vi "CD Init_Prepare Inline Data_Compute Index from CWD1 FOR Broadcast.vi"(11 "message":T1 {"Timestamp Channel Data Reference" format="%.0x"; "Status Channel Data Refs" format="%.0x"; "Words Item Refs" format="%.0x"; "Words Block Data Refs"."Data Reference" format="%.0x"}) -> (0 "RT to RT?":bool, 1 "Index 1":u32, 2 "Broadcast?":bool, 3 "Index 0":u16, 5 "CWD1.SA":i8)   [LabVIEW 2017, in "Ballard MIL-1553 Engine.lvlib"]
uses:
  Ballard MIL-1553 Engine.lvlib
  Shared/Controls and Global/RT Message.ctl
  Shared/Controls and Global/RT messageType.ctl
  Shared/Controls and Global/RT CWD1.ctl
  Shared/Controls and Global/RT CWD2.ctl
  <vilib>/NI Veristand/Custom Device API/Data Reference.ctl
  <vilib>/NI Veristand/Custom Device API/Custom Device Item Ref.ctl
  <vilib>/NI Veristand/Custom Device API/Block Data Reference.ctl
  <vilib>/NI VeriStand/Custom Device API/Custom Device API.lvlib
  Shared/Ballard 1553 Shared.lvlib
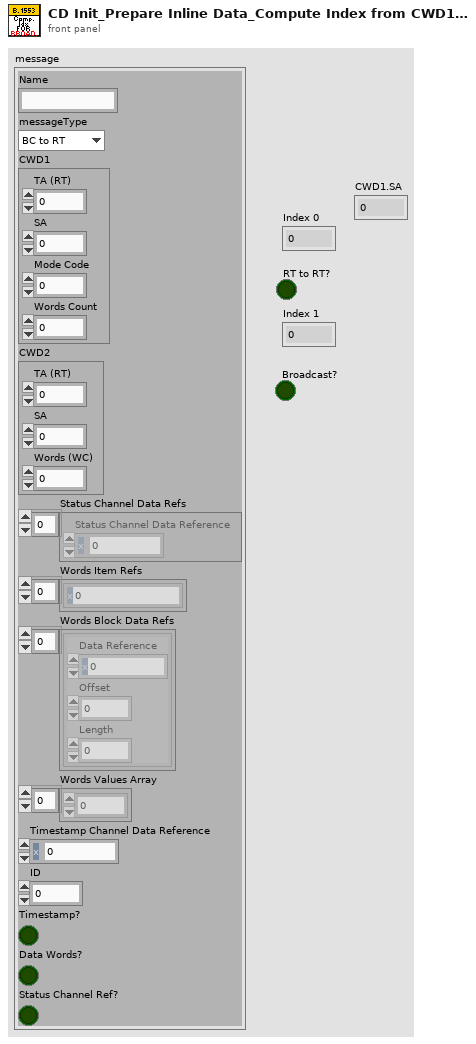
[diagram p1: front panel]
types:
  T1 = typedef "Ballard 1553 Shared.lvlib/RT Message.ctl" = cluster{"Name":string, "messageType":T2, "CWD1":T3, "CWD2":T4, "Status Channel Data Refs":T5[], "Words Item Refs":T6[], "Words Block Data Refs":T7[], "Words Values Array":u16[], "Timestamp Channel Data Reference":T5, "ID":i32, "Timestamp?":bool, "Data Words?":bool, "Status Channel Ref?":bool}
  T2 = typedef "Ballard 1553 Shared.lvlib/RT messageType.ctl" = enum16{"BC to RT", "RT to BC", "RT to RT", "MC (Rx)", "MC (Tx)"}
  T3 = typedef "Ballard 1553 Shared.lvlib/RT CWD1.ctl" = cluster{"TA (RT)":i8, "SA":i8, "Mode Code":i8, "Words Count":i8}
  T4 = typedef "Ballard 1553 Shared.lvlib/RT CWD2.ctl" = cluster{"TA (RT)":i8, "SA":i8, "Words (WC)":i8}
  T5 = typedef "Custom Device API.lvlib/Data Reference.ctl" = i32
  T6 = typedef "Custom Device API.lvlib/Custom Device Item Ref.ctl" = u64
  T7 = typedef "Custom Device API.lvlib/Block Data Reference.ctl" = cluster{"Data Reference":T5, "Offset":u64, "Length":u64}
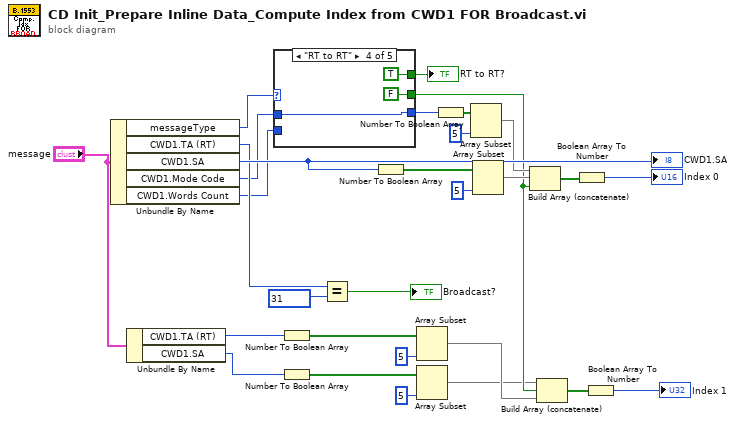
[diagram p0: block diagram]
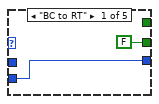
[diagram p2: hidden frame]
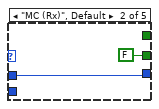
[diagram p3: hidden frame]
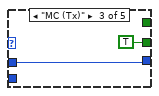
[diagram p4: hidden frame]
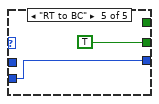
[diagram p5: hidden frame]
diagram:
  n1 = Unbundle By Name("message") -> ("messageType"=w23:T2, "CWD1.TA (RT)"=w10:i8, "CWD1.SA"=w24:i8, "CWD1.Mode Code"=w6:i8, "CWD1.Words Count"=w5:i8)
  "CWD1.SA" <- w24
  n2 = Unbundle By Name("message") -> ("CWD1.TA (RT)"=w16:i8, "CWD1.SA"=w15:i8)
  n3 = case shown="\"RT to RT\"" w23 {
    tunnel: [FALSE FALSE TRUE FALSE TRUE] -> w2
    tunnel: [_ _ _ TRUE _] -> w22
    tunnel: w6 -> [_ w32 w34 w36 _]
    tunnel: w5 -> [w30 _ _ _ w39]
    tunnel: [w30 w32 w34 w36 w39] -> w4
    frame "BC to RT" {
    }
    frame "MC (Rx)", Default {
    }
    frame "MC (Tx)" {
    }
    frame "RT to RT" {
    }
    frame "RT to BC" {
    }
  }
  "RT to RT?" <- w22
  n4 = Number To Boolean Array(number=w16) -> (Boolean array=w20:bool[])
  n5 = Number To Boolean Array(number=w15) -> (Boolean array=w19:bool[])
  n6 = Equal?(x=w10, y=i8 31) -> (x = y?=→"Broadcast?":bool)
  n7 = Number To Boolean Array(number=w24) -> (Boolean array=w26:bool[])
  n8 = Array Subset(array=w20, length=5) -> (w14:bool[])  [unwired: 1 in]
  n9 = Array Subset(array=w19, length=5) -> (w1:bool[])  [unwired: 1 in]
  n10 = Number To Boolean Array(number=w4) -> (Boolean array=w25:bool[])
  n11 = Array Subset(array=w25, length=5) -> (w7:bool[])  [unwired: 1 in]
  n12 = Array Subset(array=w26, length=5) -> (w3:bool[])  [unwired: 1 in]
  n13 = Build Array (concatenate)(w7, w3, w2) -> (w13:bool[])
  n14 = Build Array (concatenate)(w1, w2, w14) -> (w11:bool[])
  n15 = Boolean Array To Number(Boolean array=w13) -> (number=→"Index 0":u16)
  n16 = Boolean Array To Number(Boolean array=w11) -> (number=→"Index 1":u32)
